vi "log analysis_gps.vi"() -> ()   [LabVIEW 2019] (continued)
\t-1.749398\t-175.069883\t0.291000\t0.008000\n\t\n15:47:23.2\tlog_raw\tgps_raw\t#INSPVAXA,USB3,0,49.5,FINESTEERING,2107,283661.200,02000000,471d,15824;INS_ALIGNMENT_COMPLETE,INS_RTKFIXED,37.37126187130,126.72202999654,7.8827,22.3000,0.0166,-0.2769,0.0144,-0.534535443,-1.728487239,265.001971487,0.4359,0.2961,0.5778,0.1123,0.0926,0.0785,0.0961,0.1008,5.1311,0f000001,0*51cc925f\n\tsystem status\tnormal 2 27.800000 0 0\trobot status\t105.841527\t125.597807\t7.882700\t-0.534535\t-1.728487\t-175.001971\t0.284000\t0.012000\n\t\n15:47:23.7\tlog_raw\tgps_raw\t#DUALANTENNAHEADINGA,USB3,0,49.5,FINESTEERING,2107,283661.700,02000000,d426,15824;INSUFFICIENT_OBS,NONE,-1.000000000,0.000000000,0.000000000,0.0,0.000000000,0.000000000,\"631T\",12,4,4,3,04,00,20,03*15f903f8\n\tsystem status\tnormal 2 27.800000 0 0\trobot status\t105.702965\t125.590854\t7.884200\t-0.871076\t-0.905355\t-174.823029\t0.389000\t-0.120000\n\t\n15:47:24.2\tlog_raw\tgps_raw\t#DUALANTENNAHEADINGA,USB3,0,48.0,FINESTEERING,2107,283662.200,02000000,d426,15824;INSUFFICIENT_OBS,NONE,-1.000000000,0.000000000,0.000000000,0.0,0.000000000,0.000000000,\"631T\",12,4,4,3,04,00,20,03*45bc2fa2\n\tsystem status\tnormal 2 27.800000 0 0\trobot status\t105.562658\t125.586822\t7.884400\t-0.819819\t-0.206414\t-174.816486\t0.286000\t0.006000\n\t\n15:47:24.7\tlog_raw\tgps_raw\t#INSPVAXA,USB3,0,48.0,FINESTEERING,2107,283662.700,02000000,471d,15824;INS_ALIGNMENT_COMPLETE,INS_RTKFIXED,37.37126171572,126.72202522799,7.8823,22.3000,-0.0067,-0.2635,0.0136,-1.179961552,0.094212856,265.044425368,0.4362,0.2961,0.5779,0.1131,0.0926,0.0785,0.0961,0.1008,5.1327,0f000001,0*9a1b8d6f\n\tsystem status\tnormal 2 27.900000 0 0\trobot status\t105.419137\t125.580546\t7.882300\t-1.179962\t0.094213\t-175.044425\t0.278000\t0.003000\n\t\n15:47:25.2\tlog_raw\tgps_raw\t#DUALANTENNAHEADINGA,USB3,0,49.0,FINESTEERING,2107,283663.200,02000000,d426,15824;INSUFFICIENT_OBS,NONE,-1.000000000,0.000000000,0.000000000,0.0,0.000000000,0.000000000,\"631T\",12,4,4,3,04,00,20,03*4c20fddf\n\tsystem status\tnormal 2 27.900000 0 0\trobot status\t105.284116\t125.575156\t7.883700\t-1.526473\t0.492436\t-175.160100\t0.292000\t-0.033000\n\t\n15:47:25.7\tlog_raw\tgps_raw\t#DUALANTENNAHEADINGA,USB3,0,49.0,FINESTEERING,2107,283663.700,02000000,d426,15824;INSUFFICIENT_OBS,NONE,-1.000000000,0.000000000,0.000000000,0.0,0.000000000,0.000000000,\"631T\",13,4,4,3,04,00,20,03*4cd16cde\n\tsystem status\tnormal 2 27.900000 0 0\trobot status\t105.149860\t125.571077\t7.886600\t-1.585695\t1.181553\t-175.183100\t0.294000\t-0.020000\n\t\n15:47:26.2\tlog_raw\tgps_raw\t#DUALANTENNAHEADINGA,USB3,0,53.0,FINESTEERING,2107,283664.200,02000000,d426,15824;INSUFFICIENT_OBS,NONE,-1.000000000,0.000000000,0.000000000,0.0,0.000000000,0.000000000,\"631T\",14,4,4,3,04,00,20,02*f110e9d9\n\tsystem status\tnormal 2 27.800000 0 0\trobot status\t105.010520\t125.564554\t7.892600\t-1.984977\t1.172369\t-175.175072\t0.296000\t-0.009000\n\t\n15:47:26.7\tlog_raw\tgps_raw\t#DUALANTENNAHEADINGA,USB3,0,53.0,FINESTEERING,2107,283664.700,02000000,d426,15824;INSUFFICIENT_OBS,NONE,-1.000000000,0.000000000,0.000000000,0.0,0.000000000,0.000000000,\"631T\",15,4,4,3,04,00,20,02*f1e178d8\n\tsystem status\tnormal 2 27.900000 0 0\trobot status\t104.866280\t125.562759\t7.898100\t-1.643568\t1.568433\t-175.385137\t0.303000\t-0.018000\n\t\n15:47:27.2\tlog_raw\tgps_raw\t#DUALANTENNAHEADINGA,USB3,0,50.0,FINESTEERING,2107,283665.200,02000000,d426,15824;INSUFFICIENT_OBS,NONE,-1.000000000,0.000000000,0.000000000,0.0,0.000000000,0.000000000,\"631T\",13,4,4,3,04,00,20,03*0d3c2d31\n\tsystem status\tnormal 2 27.900000 0 0\trobot status\t104.717899\t125.556202\t7.901900\t-2.175035\t2.158905\t-175.701482\t0.303000\t-0.049000\n\t\n15:47:27.7\tlog_raw\tgps_raw\t#DUALANTENNAHEADINGA,USB3,0,50.0,FINESTEERING,2107,283665.700,02000000,d426,15824;INSUFFICIENT_OBS,NONE,-1.000000000,0.000000000,0.000000000,0.0,0.000000000,0.000000000,\"631T\",12,4,4,3,04,00,20,02*7aca8ca6\n\tsystem status\tnormal 2 27.800000 0 0\trobot status\t104.573395\t125.553571\t7.908800\t-2.110560\t2.141372\t-176.036510\t0.311000\t-0.034000\n\t\n15:47:28.2\tlog_raw\tgps_raw\t#DUALANTENNAHEADINGA,USB3,0,49.5,FINESTEERING,2107,283666.200,02000000,d426,15824;INSUFFICIENT_OBS,NONE,-1.000000000,0.000000000,0.000000000,0.0,0.000000000,0.000000000,\"631T\",12,4,4,3,04,00,20,03*18930aef\n\tsystem status\tnormal 2 27.800000 0 0\trobot status\t104.418430\t125.550188\t7.915100\t-2.269862\t2.122656\t-176.495930\t0.394000\t0.113000\n\t\n15:47:28.7\tlog_raw\tgps_raw\t\tsystem status\tnormal 2 27.800000 0 0\trobot status\t104.271361\t125.550531\t7.920700\t-2.130480\t1.933923\t-177.098669\t0.402000\t0.141000\n\t\n15:47:29.2\tlog_raw\tgps_raw\t#DUALANTENNAHEADINGA,USB3,0,51.0,FINESTEERING,2107,283667.200,02000000,d426,15824;INSUFFICIENT_OBS,NONE,-1.000000000,0.000000000,0.000000000,0.0,0.000000000,0.000000000,\"631T\",14,4,4,3,04,00,20,03*f8f6796c\n\tsystem status\tnormal 2 27.700000 0 0\trobot status\t104.125597\t125.551980\t7.926900\t-2.197035\t1.911660\t-177.915300\t0.350000\t0.055000\n\t\n15:47:29.7\tlog_raw\tgps_raw\t#DUALANTENNAHEADINGA,USB3,0,51.0,FINESTEERING,2107,283667.700,02000000,d426,15824;INSUFFICIENT_OBS,NONE,-1.000000000,0.000000000,0.000000000,0.0,0.000000000,0.000000000,\"631T\",14,4,4,3,04,00,20,02*58e258a3\n\tsystem status\tnormal 2 27.700000 0 0\trobot status\t103.980327\t125.554709\t7.933500\t-2.393208\t1.875693\t-178.717408\t0.289000\t-0.036000\n\t\n15:47:30.2\tlog_raw\tgps_raw\t#DUALANTENNAHEADINGA,USB3,0,51.5,FINESTEERING,2107,283668.200,02000000,d426,15824;INSUFFICIENT_OBS,NONE,-1.000000000,0.000000000,0.000000000,0.0,0.000000000,0.000000000,\"631T\",13,4,4,3,04,00,20,03*e5e926ef\n\tsystem status\tnormal 2 27.800000 0 0\trobot status\t103.834212\t125.563002\t7.939200\t-2.024919\t1.603029\t-179.561928\t0.229000\t-0.114000\n\t\n15:47:30.7\tlog_raw\tgps_raw\t#DUALANTENNAHEADINGA,USB3,0,51.5,FINESTEERING,2107,283668.700,02000000,d426,15824;INSUFFICIENT_OBS,NONE,-1.000000000,0.000000000,0.000000000,0.0,0.000000000,0.000000000,\"631T\",12,4,4,3,04,00,20,03*e518b7ee\n\tsystem status\tnormal 2 27.800000 0 0\trobot status\t103.706860\t125.571273\t7.943700\t-1.912750\t1.464702\t179.878930\t0.099000\t-0.005000\n\t\n15:47:31.2\tlog_raw\tgps_raw\t#DUALANTENNAHEADINGA,USB3,0,49.0,FINESTEERING,2107,283669.200,02000000,d426,15824;INSUFFICIENT_OBS,NONE,-1.000000000,0.000000000,0.000000000,0.0,0.000000000,0.000000000,\"631T\",12,4,4,3,04,00,20,03*4fb2de27\n\tsystem status\tnormal 2 27.800000 0 0\trobot status\t103.578139\t125.580373\t7.945800\t-2.015025\t1.317294\t179.548370\t0.270000\t-0.089000\n\t\n15:47:31.7\tlog_raw\tgps_raw\t#DUALANTENNAHEADINGA,USB3,0,49.0,FINESTEERING,2107,283669.700,02000000,d426,15824;INSUFFICIENT_OBS,NONE,-1.000000000,0.000000000,0.000000000,0.0,0.000000000,0.000000000,\"631T\",12,4,4,3,04,00,20,02*efa6ffe8\n\tsystem status\tnormal 2 27.800000 0 0\trobot status\t103.443389\t125.589391\t7.947800\t-2.168646\t1.038797\t179.383085\t0.315000\t0.000000\n\t\n15:47:32.2\tlog_raw\tgps_raw\t#DUALANTENNAHEADINGA,USB3,0,50.0,FINESTEERING,2107,283670.200,02000000,d426,15824;INSUFFICIENT_OBS,NONE,-1.000000000,0.000000000,0.000000000,0.0,0.000000000,0.000000000,\"631T\",12,4,4,3,04,00,20,03*24750ee1\n\tsystem status\tnormal 2 27.800000 0 0\trobot status\t103.309611\t125.601920\t7.951600\t-1.888949\t0.915016\t179.178170\t0.304000\t0.012000\n\t\n15:47:32.7\tlog_raw\tgps_raw\t#DUALANTENNAHEADINGA,USB3,0,50.0,FINESTEERING,2107,283670.700,02000000,d426,15824;INSUFFICIENT_OBS,NONE,-1.000000000,0.000000000,0.000000000,0.0,0.000000000,0.000000000,\"631T\",13,4,4,3,04,00,20,03*24849fe0\n\tsystem status\tnormal 2 27.900000 0 0\trobot status\t103.174226\t125.616514\t7.954700\t-1.437536\t0.949843\t179.107263\t0.291000\t0.026000\n\t\n15:47:33.2\tlog_raw\tgps_raw\t#DUALANTENNAHEADINGA,USB3,0,50.0,FINESTEERING,2107,283671.200,02000000,d426,15824;INSUFFICIENT_OBS,NONE,-1.000000000,0.000000000,0.000000000,0.0,0.000000000,0.000000000,\"631T\",13,4,4,3,04,00,20,02*e948baf6\n\tsystem status\tnormal 2 27.800000 0 0\trobot status\t103.027425\t125.628258\t7.958900\t-1.451100\t0.751950\t179.111320\t0.296000\t0.032000\n\t\n15:47:33.7\tlog_raw\tgps_raw\t#DUALANTENNAHEADINGA,USB3,0,50.0,FINESTEERING,2107,283671.700,02000000,d426,15824;INSUFFICIENT_OBS,NONE,-1.000000000,0.000000000,0.000000000,0.0,0.000000000,0.000000000,\"631T\",12,4,4,3,04,00,20,02*e9b92bf7\n\tsystem status\tnormal 2 27.900000 0 0\trobot status\t102.871613\t125.638877\t7.960600\t-1.577622\t0.823494\t179.153845\t0.306000\t0.029000\n\t\n15:47:34.2\tlog_raw\tgps_raw\t#DUALANTENNAHEADINGA,USB3,0,47.5,FINESTEERING,2107,283672.200,02000000,d426,15824;INSUFFICIENT_OBS,NONE,-1.000000000,0.000000000,0.000000000,0.0,0.000000000,0.000000000,\"631T\",13,4,4,3,04,00,20,03*4a2d65dd\n\tsystem status\tnormal 2 27.800000 0 0\trobot status\t102.727478\t125.652101\t7.963400\t-1.336233\t0.876198\t179.513411\t0.340000\t-0.041000\n\t\n15:47:34.7\tlog_raw\tgps_raw\t#DUALANTENNAHEADINGA,USB3,0,47.5,FINESTEERING,2107,283672.700,02000000,d426,15824;INSUFFICIENT_OBS,NONE,-1.000000000,0.000000000,0.000000000,0.0,0.000000000,0.000000000,\"631T\",11,4,4,3,04,00,20,03*e98a7275\n\tsystem status\tnormal 2 27.700000 0 0\trobot status\t102.584118\t125.664970\t7.965600\t-1.001130\t0.865934\t-179.684360\t0.289000\t0.047000\n\t\n15:47:35.2\tlog_raw\tgps_raw\t#DUALANTENNAHEADINGA,USB3,0,49.0,FINESTEERING,2107,283673.200,02000000,d426,15824;INSUFFICIENT_OBS,NONE,-1.000000000,0.000000000,0.000000000,0.0,0.000000000,0.000000000,\"631T\",12,4,4,3,04,00,20,02*c4457f3d\n\tsystem status\tnormal 2 27.500000 0 0\trobot status\t102.442950\t125.672792\t7.967600\t-1.200080\t0.869619\t-178.506958\t0.290000\t0.033000\n\t\n15:47:35.7\tlog_raw\tgps_raw\t#DUALANTENNAHEADINGA,USB3,0,49.0,FINESTEERING,2107,283673.700,02000000,d426,15824;INSUFFICIENT_OBS,NONE,-1.000000000,0.000000000,0.000000000,0.0,0.000000000,0.000000000,\"631T\",13,4,4,3,04,00,20,03*b3b3deaa\n\tsystem status\tnormal 2 27.400000 0 0\trobot status\t102.301599\t125.675630\t7.970100\t-1.366627\t0.503237\t-176.945977\t0.292000\t0.049000\n\t\n15:47:36.2\tlog_raw\tgps_raw\t#DUALANTENNAHEADINGA,USB3,0,50.0,FINESTEERING,2107,283674.200,02000000,d426,15824;INSUFFICIENT_OBS,NONE,-1.000000000,0.000000000,0.000000000,0.0,0.000000000,0.000000000,\"631T\",13,4,4,3,04,00,20,03*9f869b9c\n\tsystem status\tnormal 2 27.400000 0 0\trobot status\t102.163674\t125.676713\t7.974400\t-1.299675\t0.317092\t-175.226146\t0.304000\t0.058000\n\t\n15:47:36.7\tlog_raw\tgps_raw\t#INSPVAXA,USB3,0,50.0,FINESTEERING,2107,283674.750,02000000,471d,15824;INS_ALIGNMENT_COMPLETE,INS_RTKFIXED,37.37126252882,126.72198672229,7.9795,22.3000,-0.0186,-0.2998,0.0327,-1.236759140,0.298585225,263.242315357,0.4398,0.2975,0.5789,0.1131,0.0929,0.0786,0.0960,0.1008,5.0828,0f000001,0*30bc741b\n\tsystem status\tnormal 2 27.400000 0 0\trobot status\t102.008365\t125.670829\t7.979500\t-1.236759\t0.298585\t-173.242315\t0.310000\t0.068000\n\t\n15:47:37.2\tlog_raw\tgps_raw\t#DUALANTENNAHEADINGA,USB3,0,47.5,FINESTEERING,2107,283675.200,02000000,d426,15824;INSUFFICIENT_OBS,NONE,-1.000000000,0.000000000,0.000000000,0.0,0.000000000,0.000000000,\"631T\",12,4,4,3,04,00,20,02*30b1cd5d\n\tsystem status\tnormal 2 27.500000 0 0\trobot status\t101.881157\t125.662058\t7.983600\t-1.357425\t0.105413\t-171.884770\t0.302000\t0.058000\n\t\n15:47:37.7\tlog_raw\tgps_raw\t#DUALANTENNAHEADINGA,USB3,0,47.5,FINESTEERING,2107,283675.700,02000000,d426,15824;INSUFFICIENT_OBS,NONE,-1.000000000,0.000000000,0.000000000,0.0,0.000000000,0.000000000,\"631T\",13,4,4,3,04,00,20,03*47476cca\n\tsystem status\tnormal 2 27.500000 0 0\trobot status\t101.741807\t125.649863\t7.985900\t-1.401248\t0.156405\t-170.535957\t0.300000\t0.034000\n\t\n15:47:38.2\tlog_raw\tgps_raw\t#DUALANTENNAHEADINGA,USB3,0,50.0,FINESTEERING,2107,283676.200,02000000,d426,15824;INSUFFICIENT_OBS,NONE,-1.000000000,0.000000000,0.000000000,0.0,0.000000000,0.000000000,\"631T\",13,4,4,3,04,00,20,02*3331a2b8\n\tsystem status\tnormal 2 27.500000 0 0\trobot status\t101.602528\t125.635550\t7.989300\t-1.281281\t0.182913\t-169.273550\t0.304000\t0.035000\n\t\n15:47:38.7\tlog_raw\tgps_raw\t#INSPVAXA,USB3,0,50.0,FINESTEERING,2107,283676.750,02000000,471d,15824;INS_ALIGNMENT_COMPLETE,INS_RTKFIXED,37.37126202802,126.72198037867,7.9931,22.3000,-0.0270,-0.2983,0.0289,-1.276938431,0.174085147,258.154591337,0.4371,0.2976,0.5788,0.1128,0.0927,0.0785,0.0959,0.1007,5.0828,0f000001,0*1eb9a34f\n\tsystem status\tnormal 2 27.500000 0 0\trobot status\t101.446458\t125.615255\t7.993100\t-1.276938\t0.174085\t-168.154591\t0.309000\t0.036000\n\t\n15:47:39.2\tlog_raw\tgps_raw\t#INSPVAXA,USB3,0,47.5,FINESTEERING,2107,283677.250,02000000,471d,15824;INS_ALIGNMENT_COMPLETE,INS_RTKFIXED,37.37126184306,126.72197878066,7.9954,22.3000,-0.0249,-0.2800,0.0095,-1.329008924,0.068233484,257.455385518,0.4363,0.2976,0.5789,0.1128,0.0926,0.0785,0.0959,0.1006,5.0823,0f000001,0*a0488656\n\tsystem status\tnormal 2 27.700000 0 0\trobot status\t101.304909\t125.594729\t7.995400\t-1.329009\t0.068233\t-167.455386\t0.294000\t0.024000\n\t\n15:47:39.7\tlog_raw\tgps_raw\t\tsystem status\tnormal 2 27.700000 0 0\trobot status\t101.178617\t125.576497\t7.997000\t-1.321443\t0.121377\t-166.935462\t0.272000\t0.053000\n\t\n15:47:40.2\tlog_raw\tgps_raw\t\tsystem status\tnormal 2 27.600000 0 0\trobot status\t101.060799\t125.559123\t7.999900\t-1.339962\t0.318685\t-166.437151\t0.256000\t0.107000\n\t\n15:47:40.7\tlog_raw\tgps_raw\t#INSPVAXA,USB3,0,44.5,FINESTEERING,2107,283678.750,02000000,471d,15824;INS_ALIGNMENT_COMPLETE,INS_RTKFIXED,37.37126126052,126.72197417876,8.0025,22.3000,-0.0388,-0.3139,0.0075,-1.341441151,0.143163163,255.994609032,0.4352,0.2975,0.5790,0.1123,0.0928,0.0785,0.0959,0.1006,5.0816,0f000001,0*2dcb75ae\n\tsystem status\tnormal 2 27.700000 0 0\trobot status\t100.897280\t125.530081\t8.002500\t-1.341441\t0.143163\t-165.994609\t0.230000\t0.123000\n\t\n15:47:41.2\tlog_raw\tgps_raw\t#INSPVAXA,USB3,0,50.0,FINESTEERING,2107,283679.250,02000000,471d,15824;INS_ALIGNMENT_COMPLETE,INS_RTKFIXED,37.37126102386,126.72197256335,8.0029,22.3000,-0.0378,-0.3051,0.0239,-1.252291621,0.317106039,255.710782643,0.4355,0.2977,0.5792,0.1125,0.0927,0.0786,0.0959,0.1006,5.0819,0f000001,0*497f861f\n\tsystem status\tnormal 2 27.800000 0 0\trobot status\t100.754189\t125.503817\t8.002900\t-1.252292\t0.317106\t-165.710783\t0.206000\t0.142000\n\t\n15:47:41.7\tlog_raw\tgps_raw\t#DUALANTENNAHEADINGA,USB3,0,50.0,FINESTEERING,2107,283679.700,02000000,d426,15824;INSUFFICIENT_OBS,NONE,-1.000000000,0.000000000,0.000000000,0.0,0.000000000,0.000000000,\"631T\",13,4,4,3,04,00,20,03*917eb173\n\tsystem status\tnormal 2 27.800000 0 0\trobot status\t100.626127\t125.478833\t8.004200\t-1.300155\t0.357436\t-165.554866\t0.246000\t0.082000\n\t\n15:47:42.2\tlog_raw\tgps_raw\t#INSPVAXA,USB3,0,49.5,FINESTEERING,2107,283680.250,02000000,471d,15824;INS_ALIGNMENT_COMPLETE,INS_RTKFIXED,37.37126052998,126.72196935056,8.0055,22.3000,-0.0369,-0.2979,0.0271,-1.221523222,0.248269535,255.390291305,0.4350,0.2975,0.5791,0.1126,0.0927,0.0786,0.0959,0.1006,5.0824,0f000001,0*4c9222e8\n\tsystem status\tnormal 2 27.800000 0 0\trobot status\t100.469606\t125.449008\t8.005500\t-1.221523\t0.248270\t-165.390291\t0.265000\t0.060000\n\t\n15:47:42.7\tlog_raw\tgps_raw\t#INSPVAXA,USB3,0,49.5,FINESTEERING,2107,283680.750,02000000,471d,15824;INS_ALIGNMENT_COMPLETE,INS_RTKFIXED,37.37126029067,126.72196774054,8.0075,22.3000,-0.0484,-0.2930,0.0156,-1.123777574,0.215686141,255.306454627,0.4350,0.2975,0.5791,0.1126,0.0927,0.0786,0.0959,0.1006,5.0824,0f000001,0*b1d08eab\n\tsystem status\tnormal 2 27.800000 0 0\trobot status\t100.326993\t125.422450\t8.007500\t-1.123778\t0.215686\t-165.306455\t0.353000\t-0.070000\n\t\n15:47:43.2\tlog_raw\tgps_raw\t#DUALANTENNAHEADINGA,USB3,0,47.5,FINESTEERING,2107,283681.200,02000000,d426,15824;INSUFFICIENT_OBS,NONE,-1.000000000,0.000000000,0.000000000,0.0,0.000000000,0.000000000,\"631T\",13,4,4,3,04,00,20,02*8c2dc70b\n\tsystem status\tnormal 2 27.800000 0 0\trobot status\t100.200318\t125.396716\t8.008600\t-1.364227\t0.259230\t-165.309745\t0.296000\t0.001000\n\t\n15:47:43.7\tlog_raw\tgps_raw\t#DUALANTENNAHEADINGA,USB3,0,47.5,FINESTEERING,2107,283681.700,02000000,d426,15824;INSUFFICIENT_OBS,NONE,-1.000000000,0.000000000,0.000000000,0.0,0.000000000,0.000000000,\"631T\",13,4,4,3,04,00,20,03*2c39e6c4\n\tsystem status\tnormal 2 27.800000 0 0\trobot status\t100.058386\t125.369198\t8.010200\t-1.337236\t0.106302\t-165.240050\t0.349000\t-0.071000\n\t\n15:47:44.2\tlog_raw\tgps_raw\t#DUALANTENNAHEADINGA,USB3,0,53.0,FINESTEERING,2107,283682.200,02000000,d426,15824;INSUFFICIENT_OBS,NONE,-1.000000000,0.000000000,0.000000000,0.0,0.000000000,0.000000000,\"631T\",13,4,4,3,04,00,20,02*f482535a\n\tsystem status\tnormal 2 27.800000 0 0\trobot status\t99.916585\t125.340598\t8.012100\t-1.398981\t0.149147\t-165.140056\t0.293000\t0.019000\n\t\n15:47:44.7\tlog_raw\tgps_raw\t#INSPVAXA,USB3,0,53.0,FINESTEERING,2107,283682.750,02000000,471d,15824;INS_ALIGNMENT_COMPLETE,INS_RTKFIXED,37.37125926494,126.72196137618,8.0142,22.3000,-0.0531,-0.2940,0.0193,-1.467222683,0.192661373,255.088191975,0.4346,0.2973,0.5792,0.1126,0.0928,0.0786,0.0959,0.1005,5.0834,0f000001,0*e49cbeff\n\tsystem status\tnormal 2 27.800000 0 0\trobot status\t99.763248\t125.308616\t8.014200\t-1.467223\t0.192661\t-165.088192\t0.352000\t-0.079000\n\t\n15:47:45.2\tlog_raw\tgps_raw\t#DUALANTENNAHEADINGA,USB3,0,51.5,FINESTEERING,2107,283683.200,02000000,d426,15824;INSUFFICIENT_OBS,NONE,-1.000000000,0.000000000,0.000000000,0.0,0.000000000,0.000000000,\"631T\",13,4,4,3,04,00,20,03*73ae2c91\n\tsystem status\tnormal 2 27.800000 0 0\trobot status\t99.634729\t125.283250\t8.015500\t-1.390828\t0.179060\t-165.064944\t0.292000\t0.016000\n\t\n15:47:45.7\tlog_raw\tgps_raw\t#INSPVAXA,USB3,0,51.5,FINESTEERING,2107,283683.750,02000000,471d,15824;INS_ALIGNMENT_COMPLETE,INS_RTKFIXED,37.37125874592,126.72195815928,8.0147,22.3000,-0.0440,-0.2967,0.0132,-1.341050050,-0.067435832,254.924614252,0.4345,0.2971,0.5791,0.1126,0.0928,0.0785,0.0959,0.1005,5.0840,0f000001,0*701f89f0\n\tsystem status\tnormal 2 27.800000 0 0\trobot status\t99.478300\t125.251016\t8.014700\t-1.341050\t-0.067436\t-164.924614\t0.429000\t-0.182000\n\t\n15:47:46.2\tlog_raw\tgps_raw\t#DUALANTENNAHEADINGA,USB3,0,52.0,FINESTEERING,2107,283684.200,02000000,d426,15824;INSUFFICIENT_OBS,NONE,-1.000000000,0.000000000,0.000000000,0.0,0.000000000,0.000000000,\"631T\",13,4,4,3,04,00,20,02*27679969\n\tsystem status\tnormal 2 27.800000 0 0\trobot status\t99.351672\t125.225493\t8.015100\t-1.339484\t-0.170891\t-164.827826\t0.237000\t0.097000\n\t\n15:47:46.7\tlog_raw\tgps_raw\t#INSPVAXA,USB3,0,52.0,FINESTEERING,2107,283684.750,02000000,471d,15824;INS_ALIGNMENT_COMPLETE,INS_RTKFIXED,37.37125823226,126.72195499542,8.0159,22.3000,-0.0425,-0.2912,0.0233,-1.481512417,-0.232627459,254.717814630,0.4345,0.2970,0.5790,0.1126,0.0928,0.0785,0.0959,0.1005,5.0847,0f000001,0*bc004070\n\tsystem status\tnormal 2 27.800000 0 0\trobot status\t99.198051\t125.194011\t8.015900\t-1.481512\t-0.232627\t-164.717815\t0.430000\t-0.193000\n\t\n15:47:47.2\tlog_raw\tgps_raw\t#DUALANTENNAHEADINGA,USB3,0,54.0,FINESTEERING,2107,283685.200,02000000,d426,15824;INSUFFICIENT_OBS,NONE,-1.000000000,0.000000000,0.000000000,0.0,0.000000000,0.000000000,\"631T\",13,4,4,3,04,00,20,03*bf535cbf\n\tsystem status\tnormal 2 27.800000 0 0\trobot status\t99.072052\t125.168405\t8.017800\t-1.521026\t-0.355699\t-164.511817\t0.245000\t0.084000\n\t\n15:47:47.7\tlog_raw\tgps_raw\t#DUALANTENNAHEADINGA,USB3,0,54.0,FINESTEERING,2107,283685.700,02000000,d426,15824;INSUFFICIENT_OBS,NONE,-1.000000000,0.000000000,0.000000000,0.0,0.000000000,0.000000000,\"631T\",15,4,4,3,04,00,20,03*f59c46f5\n\tsystem status\tnormal 2 27.800000 0 0\trobot status\t98.933125\t125.139867\t8.018400\t-1.376883\t-0.262136\t-164.273849\t0.254000\t0.072000\n\t\n15:47:48.2\tlog_raw\tgps_raw\t#INSPVAXA,USB3,0,47.0,FINESTEERING,2107,283686.250,02000000,471d,15824;INS_ALIGNMENT_COMPLETE,INS_RTKFIXED,37.37125745168,126.72195028422,8.0177,22.3000,-0.0421,-0.2788,0.0295,-1.327379585,-0.197998940,254.015433265,0.4342,0.2970,0.5788,0.1125,0.0928,0.0785,0.0959,0.1004,5.0859,0f000001,0*059a606c\n\tsystem status\tnormal 2 27.800000 0 0\trobot status\t98.780741\t125.107384\t8.017700\t-1.327380\t-0.197999\t-164.015433\t0.374000\t-0.106000\n\t\n15:47:48.7\tlog_raw\tgps_raw\t#INSPVAXA,USB3,0,47.0,FINESTEERING,2107,283686.750,02000000,471d,15824;INS_ALIGNMENT_COMPLETE,INS_RTKFIXED,37.37125719652,126.72194873669,8.0201,22.3000,-0.0424,-0.2865,0.0311,-1.155721868,-0.143426026,253.623399398,0.4342,0.2970,0.5788,0.1125,0.0928,0.0785,0.0959,0.1004,5.0859,0f000001,0*874a06ff\n\tsystem status\tnormal 2 27.800000 0 0\trobot status\t98.643663\t125.079067\t8.020100\t-1.155722\t-0.143426\t-163.623399\t0.285000\t0.042000\n\t\n15:47:49.2\tlog_raw\tgps_raw\t#INSPVAXA,USB3,0,48.5,FINESTEERING,2107,283687.250,02000000,471d,15824;INS_ALIGNMENT_COMPLETE,INS_RTKFIXED,37.37125692308,126.72194717786,8.0216,22.3000,-0.0335,-0.2418,0.0315,-1.192319582,-0.154191109,253.231237079,0.4341,0.2971,0.5788,0.1124,0.0928,0.0785,0.0959,0.1004,5.0866,0f000001,0*54818d56\n\tsystem status\tnormal 2 27.700000 0 0\trobot status\t98.505584\t125.048721\t8.021600\t-1.192320\t-0.154191\t-163.231237\t0.319000\t-0.041000\n\t\n15:47:49.7\tlog_raw\tgps_raw\t\tsystem status\tnormal 2 27.700000 0 0\trobot status\t98.411193\t125.029187\t8.022300\t-1.203648\t0.044720\t-163.074738\t0.395000\t-0.024000\n\t\n15:47:50.2\tlog_raw\tgps_raw\t#INSPVAXA,USB3,0,48.0,FINESTEERING,2107,283688.250,02000000,471d,15824;INS_ALIGNMENT_COMPLETE,INS_RTKFIXED,37.37125642172,126.72194437677,8.0235,22.3000,-0.0500,-0.3046,0.0059,-1.164662178,-0.014385646,252.588332690,0.4343,0.2973,0.5789,0.1124,0.0928,0.0785,0.0959,0.1004,5.0876,0f000001,0*78a62f40\n\tsystem status\tnormal 2 27.700000 0 0\trobot status\t98.257468\t124.993080\t8.023500\t-1.164662\t-0.014386\t-162.588333\t0.345000\t-0.033000\n\t\n15:47:50.7\tlog_raw\tgps_raw\t#INSPVAXA,USB3,0,48.0,FINESTEERING,2107,283688.750,02000000,471d,15824;INS_ALIGNMENT_COMPLETE,INS_RTKFIXED,37.37125610282,126.72194283979,8.0244,22.3000,-0.0543,-0.2923,0.0224,-1.111219856,-0.008949492,252.070206998,0.4343,0.2973,0.5789,0.1124,0.0928,0.0785,0.0959,0.1004,5.0876,0f000001,0*c44a5f5d\n\tsystem status\tnormal 2 27.700000 0 0\trobot status\t98.121325\t124.957689\t8.024400\t-1.111220\t-0.008949\t-162.070207\t0.361000\t-0.068000\n\t\n15:47:51.2\tlog_raw\tgps_raw\t#INSPVAXA,USB3,0,50.0,FINESTEERING,2107,283689.250,02000000,471d,15824;INS_ALIGNMENT_COMPLETE,INS_RTKFIXED,37.37125577091,126.72194129043,8.0250,22.3000,-0.0553,-0.2846,0.0299,-1.126484070,-0.034453614,251.571777713,0.4347,0.2976,0.5789,0.1123,0.0927,0.0785,0.0959,0.1004,5.0890,0f000001,0*4752c184\n\tsystem status\tnormal 2 27.800000 0 0\trobot status\t97.984085\t124.920853\t8.025000\t-1.126484\t-0.034454\t-161.571778\t0.264000\t0.067000\n\t\n15:47:51.7\tlog_raw\tgps_raw\t#INSPVAXA,USB3,0,50.0,FINESTEERING,2107,283689.750,02000000,471d,15824;INS_ALIGNMENT_COMPLETE,INS_RTKFIXED,37.37125543079,126.72193970784,8.0254,22.3000,-0.0623,-0.2845,0.0344,-1.115085970,-0.181471482,251.113733002,0.4347,0.2976,0.5789,0.1123,0.0927,0.0785,0.0959,0.1004,5.0890,0f000001,0*e6043553\n\tsystem status\tnormal 2 27.700000 0 0\trobot status\t97.843902\t124.883107\t8.025400\t-1.115086\t-0.181471\t-161.113733\t0.347000\t-0.040000\n\t\n15:47:52.2\tlog_raw\tgps_raw\t#INSPVAXA,USB3,0,51.5,FINESTEERING,2107,283690.250,02000000,471d,15824;INS_ALIGNMENT_COMPLETE,INS_RTKFIXED,37.37125508435,126.72193816260,8.0268,22.3000,-0.0829,-0.2745,0.0314,-1.131096634,-0.362526816,250.672431743,0.4348,0.2977,0.5789,0.1123,0.0927,0.0785,0.0959,0.1004,5.0905,0f000001,0*0f3c6f4d\n\tsystem status\tnormal 2 27.700000 0 0\trobot status\t97.707027\t124.844659\t8.026800\t-1.131097\t-0.362527\t-160.672432\t0.294000\t0.018000\n\t\n15:47:52.7\tlog_raw\tgps_raw\t#INSPVAXA,USB3,0,51.5,FINESTEERING,2107,283690.750,02000000,471d,15824;INS_ALIGNMENT_COMPLETE,INS_RTKFIXED,37.37125472381,126.72193660268,8.0270,22.3000,-0.0761,-0.2693,0.0189,-1.124428932,-0.555258111,250.148936400,0.4348,0.2977,0.5789,0.1123,0.0927,0.0785,0.0959,0.1004,5.0905,0f000001,0*bccc2e0c\n\tsystem status\tnormal 2 27.700000 0 0\trobot status\t97.568852\t124.804646\t8.027000\t-1.124429\t-0.555258\t-160.148936\t0.283000\t0.041000\n\t\n15:47:53.2\tlog_raw\tgps_raw\t#INSPVAXA,USB3,0,51.0,FINESTEERING,2107,283691.250,02000000,471d,15824;INS_ALIGNMENT_COMPLETE,INS_RTKFIXED,37.37125435874,126.72193505456,8.0263,22.3000,-0.0670,-0.2696,0.0092,-1.064456242,-0.547416950,249.737681282,0.4347,0.2977,0.5789,0.1123,0.0927,0.0785,0.0959,0.1004,5.0921,0f000001,0*f2a7f55d\n\tsystem status\tnormal 2 27.700000 0 0\trobot status\t97.431722\t124.764131\t8.026300\t-1.064456\t-0.547417\t-159.737681\t0.301000\t-0.002000\n\t\n15:47:53.7\tlog_raw\tgps_raw\t#INSPVAXA,USB3,0,51.0,FINESTEERING,2107,283691.750,02000000,471d,15824;INS_ALIGNMENT_COMPLETE,INS_RTKFIXED,37.37125397017,126.72193349362,8.0255,22.3000,-0.0691,-0.2936,0.0158,-1.034003666,-0.605283129,249.246949956,0.4347,0.2977,0.5789,0.1123,0.0927,0.0785,0.0959,0.1004,5.0921,0f000001,0*27b79f83\n\tsystem status\tnormal 2 27.700000 0 0\trobot status\t97.293457\t124.721007\t8.025500\t-1.034004\t-0.605283\t-159.246950\t0.247000\t0.099000\n\t\n15:47:54.2\tlog_raw\tgps_raw\t#INSPVAXA,USB3,0,52.0,FINESTEERING,2107,283692.250,02000000,471d,15824;INS_ALIGNMENT_COMPLETE,INS_RTKFIXED,37.37125358988,126.72193199872,8.0234,22.3000,-0.0664,-0.2884,0.0105,-1.029506848,-0.448748893,248.703805210,0.4344,0.2976,0.5789,0.1123,0.0927,0.0785,0.0960,0.1004,5.0936,0f000001,0*b0abd4b9\n\tsystem status\tnormal 2 27.700000 0 0\trobot status\t97.161041\t124.678802\t8.023400\t-1.029507\t-0.448749\t-158.703805\t0.229000\t0.121000\n\t\n15:47:54.7\tlog_raw\tgps_raw\t#INSPVAXA,USB3,0,52.0,FINESTEERING,2107,283692.750,02000000,471d,15824;INS_ALIGNMENT_COMPLETE,INS_RTKFIXED,37.37125319556,126.72193048668,8.0218,22.3000,-0.0721,-0.2829,0.0182,-0.873709041,-0.554913446,248.258505340,0.4344,0.2976,0.5789,0.1123,0.0927,0.0785,0.0960,0.1004,5.0936,0f000001,0*33541c24\n\tsystem status\tnormal 2 27.700000 0 0\trobot status\t97.027107\t124.635040\t8.021800\t-0.873709\t-0.554913\t-158.258505\t0.387000\t-0.130000\n\t\n15:47:55.2\tlog_raw\tgps_raw\t#INSPVAXA,USB3,0,52.0,FINESTEERING,2107,283693.250,02000000,471d,15824;INS_ALIGNMENT_COMPLETE,INS_RTKFIXED,37.37125278430,126.72192895782,8.0198,22.3000,-0.0808,-0.2833,0.0124,-0.750595920,-0.512604817,247.887825209,0.4345,0.2977,0.5790,0.1123,0.0927,0.0785,0.0960,0.1005,5.0951,0f000001,0*33503232\n\tsystem status\tnormal 2 27.700000 0 0\trobot status\t96.891683\t124.589398\t8.019800\t-0.750596\t-0.512605\t-157.887825\t0.301000\t0.008000\n\t\n15:47:55.7\tlog_raw\tgps_raw\t#INSPVAXA,USB3,0,52.0,FINESTEERING,2107,283693.750,02000000,471d,15824;INS_ALIGNMENT_COMPLETE,INS_RTKFIXED,37.37125237385,126.72192745643,8.0181,22.3000,-0.0699,-0.2766,0.0107,-0.708441706,-0.569028922,247.469165126,0.4345,0.2977,0.5790,0.1123,0.0927,0.0785,0.0960,0.1005,5.0951,0f000001,0*b12f53f8\n\tsystem status\tnormal 2 27.700000 0 0\trobot status\t96.758692\t124.543846\t8.018100\t-0.708442\t-0.569029\t-157.469165\t0.271000\t0.056000\n\t\n15:47:56.2\tlog_raw\tgps_raw\t#INSPVAXA,USB3,0,51.5,FINESTEERING,2107,283694.250,02000000,471d,15824;INS_ALIGNMENT_COMPLETE,INS_RTKFIXED,37.37125195619,126.72192597903,8.0151,22.3000,-0.0814,-0.2811,0.0110,-0.711365496,-0.463120250,247.118464084,0.4343,0.2979,0.5790,0.1123,0.0927,0.0785,0.0960,0.1005,5.0966,0f000001,0*fc596ab1\n\tsystem status\tnormal 2 27.700000 0 0\trobot status\t96.627827\t124.497494\t8.015100\t-0.711365\t-0.463120\t-157.118464\t0.244000\t0.090000\n\t\n15:47:56.7\tlog_raw\tgps_raw\t#INSPVAXA,USB3,0,51.5,FINESTEERING,2107,283694.750,02000000,471d,15824;INS_ALIGNMENT_COMPLETE,INS_RTKFIXED,37.37125151893,126.72192448231,8.0119,22.3000,-0.0800,-0.2663,0.0091,-0.771660159,-0.376939407,246.768281160,0.4343,0.2979,0.5790,0.1123,0.0927,0.0785,0.0960,0.1005,5.0966,0f000001,0*6d22b1be\n\tsystem status\tnormal 2 27.800000 0 0\trobot status\t96.495250\t124.448966\t8.011900\t-0.771660\t-0.376939\t-156.768281\t0.201000\t0.145000\n\t\n15:47:57.2\tlog_raw\tgps_raw\t#INSPVAXA,USB3,0,48.0,FINESTEERING,2107,283695.250,02000000,471d,15824;INS_ALIGNMENT_COMPLETE,INS_RTKFIXED,37.37125106123,126.72192297885,8.0100,22.3000,-0.0761,-0.2505,0.0231,-0.897100380,-0.291610583,246.370264659,0.4345,0.2982,0.5790,0.1123,0.0927,0.0785,0.0960,0.1005,5.0981,0f000001,0*3984aa9f\n\tsystem status\tnormal 2 27.700000 0 0\trobot status\t96.362076\t124.398170\t8.010000\t-0.897100\t-0.291611\t-156.370265\t0.326000\t-0.030000\n\t\n15:47:57.7\tlog_raw\tgps_raw\t#INSPVAXA,USB3,0,48.0,FINESTEERING,2107,283695.750,02000000,471d,15824;INS_ALIGNMENT_COMPLETE,INS_RTKFIXED,37.37125059397,126.72192150260,8.0095,22.3000,-0.0806,-0.2555,0.0180,-1.082975458,-0.280956917,246.024954508,0.4345,0.2982,0.5790,0.1123,0.0927,0.0785,0.0960,0.1005,5.0981,0f000001,0*61086754\n\tsystem status\tnormal 2 27.700000 0 0\trobot status\t96.231312\t124.346313\t8.009500\t-1.082975\t-0.280957\t-156.024955\t0.340000\t-0.049000\n\t\n15:47:58.2\tlog_raw\tgps_raw\t#INSPVAXA,USB3,0,48.5,FINESTEERING,2107,283696.250,02000000,471d,15824;INS_ALIGNMENT_COMPLETE,INS_RTKFIXED,37.37125013310,126.72192002149,8.0081,22.3000,-0.0880,-0.2655,0.0330,-1.084281837,-0.279647129,245.685810619,0.4346,0.2982,0.5792,0.1123,0.0927,0.0785,0.0960,0.1005,5.0996,0f000001,0*ddc3e251\n\tsystem status\tnormal 2 27.700000 0 0\trobot status\t96.100117\t124.295165\t8.008100\t-1.084282\t-0.279647\t-155.685811\t0.417000\t-0.156000\n\t\n15:47:58.7\tlog_raw\tgps_raw\t#INSPVAXA,USB3,0,48.5,FINESTEERING,2107,283696.750,02000000,471d,15824;INS_ALIGNMENT_COMPLETE,INS_RTKFIXED,37.37124978634,126.72191884253,8.0066,22.3000,0.0400,0.0236,0.0167,-1.049670935,-0.308268923,245.402478860,0.4346,0.2982,0.5792,0.1123,0.0927,0.0785,0.0960,0.1005,5.0996,0f000001,0*5343d95d\n\tsystem status\tnormal 2 27.800000 0 0\trobot status\t95.995687\t124.256681\t8.006600\t-1.049671\t-0.308269\t-155.402479\t0.058000\t0.016000\n\t\n15:47:59.2\tlog_raw\tgps_raw\t#INSPVAXA,USB3,0,49.5,FINESTEERING,2107,283697.250,02000000,471d,15824;INS_ALIGNMENT_COMPLETE,INS_RTKFIXED,37.37124936191,126.72191751580,8.0075,22.3000,-0.0790,-0.2224,0.0305,-1.160332211,-0.255386119,245.257033584,0.4348,0.2981,0.5792,0.1123,0.0927,0.0785,0.0960,0.1005,5.1012,0f000001,0*9bb241a9\n\tsystem status\tnormal 2 27.800000 0 0\trobot status\t95.878168\t124.209578\t8.007500\t-1.160332\t-0.255386\t-155.257034\t0.328000\t0.026000\n\t\n15:47:59.7\tlog_raw\tgps_raw\t#INSPVAXA,USB3,0,49.5,FINESTEERING,2107,283697.750,02000000,471d,15824;INS_ALIGNMENT_COMPLETE,INS_RTKFIXED,37.37124887882,126.72191610954,8.0072,22.3000,-0.0796,-0.2609,0.0250,-1.450872911,-0.189081024,245.072886035,0.4348,0.2981,0.5792,0.1123,0.0927,0.0785,0.0960,0.1005,5.1012,0f000001,0*ca3e42a8\n\tsystem status\tnormal 2 27.800000 0 0\trobot status\t95.753603\t124.155963\t8.007200\t-1.450873\t-0.189081\t-155.072886\t0.257000\t0.086000\n\t\n15:48:00.2\tlog_raw\tgps_raw\t#INSPVAXA,USB3,0,47.0,FINESTEERING,2107,283698.250,02000000,471d,15824;INS_ALIGNMENT_COMPLETE,INS_RTKFIXED,37.37124839401,126.72191465708,8.0076,22.3000,-0.0773,-0.2590,0.0230,-1.479636169,-0.110505972,244.843169403,0.4347,0.2979,0.5791,0.1126,0.0927,0.0785,0.0960,0.1005,5.1027,0f000001,0*0006d84b\n\tsystem status\tnormal 2 27.700000 0 0\trobot status\t95.624947\t124.102158\t8.007600\t-1.479636\t-0.110506\t-154.843169\t0.247000\t0.092000\n\t\n15:48:00.7\tlog_raw\tgps_raw\t#INSPVAXA,USB3,0,47.0,FINESTEERING,2107,283698.750,02000000,471d,15824;INS_ALIGNMENT_COMPLETE,INS_RTKFIXED,37.37124790607,126.72191317649,8.0096,22.3000,-0.0919,-0.2605,0.0162,-1.323665543,0.178775756,244.574454938,0.4347,0.2979,0.5791,0.1126,0.0927,0.0785,0.0960,0.1005,5.1027,0f000001,0*97fdd670\n\tsystem status\tnormal 2 27.800000 0 0\trobot status\t95.493799\t124.048006\t8.009600\t-1.323666\t0.178776\t-154.574455\t0.255000\t0.063000\n\t\n15:48:01.2\tlog_raw\tgps_raw\t#INSPVAXA,USB3,0,47.5,FINESTEERING,2107,283699.250,02000000,471d,15824;INS_ALIGNMENT_COMPLETE,INS_RTKFIXED,37.37124741280,126.72191168515,8.0116,22.3000,-0.0880,-0.2650,0.0236,-1.277654114,0.173050319,244.335495990,0.4352,0.2978,0.5791,0.1127,0.0927,0.0785,0.0959,0.1005,5.1036,0f000001,0*401d1919\n\tsystem status\tnormal 2 27.800000 0 0\trobot status\t95.361698\t123.993262\t8.011600\t-1.277654\t0.173050\t-154.335496\t0.326000\t-0.036000\n\t\n15:48:01.7\tlog_raw\tgps_raw\t#INSPVAXA,USB3,0,47.5,FINESTEERING,2107,283699.750,02000000,471d,15824;INS_ALIGNMENT_COMPLETE,INS_RTKFIXED,37.37124691977,126.72191021065,8.0139,22.3000,-0.0941,-0.2573,0.0260,-1.295740084,0.118148751,244.043765881,0.4352,0.2978,0.5791,0.1127,0.0927,0.0785,0.0959,0.1005,5.1036,0f000001,0*b4e001ab\n\tsystem status\tnormal 2 27.800000 0 0\trobot status\t95.231089\t123.938545\t8.013900\t-1.295740\t0.118149\t-154.043766\t0.366000\t-0.095000\n\t\n15:48:02.2\tlog_raw\tgps_raw\t#INSPVAXA,USB3,0,48.5,FINESTEERING,2107,283700.250,02000000,471d,15824;INS_ALIGNMENT_COMPLETE,INS_RTKFIXED,37.37124641299,126.72190870241,8.0157,22.3000,-0.0965,-0.2606,0.0330,-1.289006516,0.186517966,243.733079989,0.4358,0.2981,0.5791,0.1128,0.0927,0.0785,0.0959,0.1005,5.1040,0f000001,0*7b588f65\n\tsystem status\tnormal 2 27.700000 0 0\trobot status\t95.097492\t123.882302\t8.015700\t-1.289007\t0.186518\t-153.733080\t0.379000\t-0.108000\n\t\n15:48:02.7\tlog_raw\tgps_raw\t#INSPVAXA,USB3,0,48.5,FINESTEERING,2107,283700.750,02000000,471d,15824;INS_ALIGNMENT_COMPLETE,INS_RTKFIXED,37.37124591211,126.72190719117,8.0183,22.3000,-0.0934,-0.2790,0.0272,-1.230862677,0.124809038,243.414753616,0.4358,0.2981,0.5791,0.1128,0.0927,0.0785,0.0959,0.1005,5.1040,0f000001,0*24944499\n\tsystem status\tnormal 2 27.700000 0 0\trobot status\t94.963629\t123.826713\t8.018300\t-1.230863\t0.124809\t-153.414754\t0.243000\t0.106000\n\t\n15:48:03.2\tlog_raw\tgps_raw\t#INSPVAXA,USB3,0,48.0,FINESTEERING,2107,283701.250,02000000,471d,15824;INS_ALIGNMENT_COMPLETE,INS_RTKFIXED,37.37124542632,126.72190568049,8.0217,22.3000,-0.0782,-0.2571,0.0284,-0.983799928,0.018605262,242.857861412,0.4361,0.2983,0.5790,0.1125,0.0928,0.0785,0.0959,0.1004,5.1037,0f000001,0*579729be\n\tsystem status\tnormal 2 27.700000 0 0\trobot status\t94.829815\t123.772800\t8.021700\t-0.983800\t0.018605\t-152.857861\t0.262000\t0.105000\n\t\n15:48:03.7\tlog_raw\tgps_raw\t#INSPVAXA,USB3,0,48.0,FINESTEERING,2107,283701.750,02000000,471d,15824;INS_ALIGNMENT_COMPLETE,INS_RTKFIXED,37.37124504941,126.72190455554,8.0252,22.3000,-0.1066,-0.3087,0.0271,-0.874891899,0.189008715,240.527059520,0.4361,0.2983,0.5790,0.1125,0.0928,0.0785,0.0959,0.1004,5.1037,0f000001,0*9bbd18ba\n\tsystem status\tnormal 2 27.100000 0 0\trobot status\t94.730169\t123.730969\t8.025200\t-0.874892\t0.189009\t-150.527060\t0.325000\t0.146000\n\t\n15:48:04.2\tlog_raw\tgps_raw\t#INSPVAXA,USB3,0,50.5,FINESTEERING,2107,283702.250,02008000,471d,15824;INS_ALIGNMENT_COMPLETE,INS_RTKFIXED,37.37124442762,126.72190307020,8.0282,22.3000,-0.1382,-0.2404,0.0216,-0.866741092,0.060143860,235.368916733,0.4360,0.2989,0.5791,0.1125,0.0927,0.0785,0.0959,0.1004,5.1028,0f000001,0*0ab995b1\n\tsystem status\tnormal 2 27.200000 4 0\trobot status\t94.598600\t123.661962\t8.028200\t-0.866741\t0.060144\t-145.368917\t0.286000\t0.213000\n\t\n15:48:04.7\tlog_raw\tgps_raw\t#INSPVAXA,USB3,0,50.5,FINESTEERING,2107,283702.750,02008000,471d,15824;INS_ALIGNMENT_COMPLETE,INS_RTKFIXED,37.37124370430,126.72190170598,8.0314,22.3000,-0.1609,-0.2382,0.0230,-1.064164970,-0.109212362,230.360783935,0.4360,0.2989,0.5791,0.1125,0.0927,0.0785,0.0959,0.1004,5.1028,0f000001,0*391c17ea\n\tsystem status\tnormal 2 27.100000 4 0\trobot status\t94.477760\t123.581686\t8.031400\t-1.064165\t-0.109212\t-140.360784\t0.321000\t0.132000\n\t\n15:48:05.2\tlog_raw\tgps_raw\t#INSPVAXA,USB3,0,50.5,FINESTEERING,2107,283703.250,02008000,471d,15824;INS_ALIGNMENT_COMPLETE,INS_RTKFIXED,37.37124291299,126.72190041379,8.0333,22.3000,-0.1952,-0.2293,0.0238,-0.984755093,-0.132867348,225.970025862,0.4356,0.2991,0.5791,0.1126,0.0928,0.0785,0.0959,0.1003,5.0999,0f000001,0*698b4567\n\tsystem status\tnormal 2 27.200000 4 0\trobot status\t94.363300\t123.493864\t8.033300\t-0.984755\t-0.132867\t-135.970026\t0.306000\t0.142000\n\t\n15:48:05.7\tlog_raw\tgps_raw\t#INSPVAXA,USB3,0,50.5,FINESTEERING,2107,283703.750,02008000,471d,15824;INS_ALIGNMENT_COMPLETE,INS_RTKFIXED,37.37124204915,126.72189921350,8.0352,22.3000,-0.1844,-0.2111,0.0260,-0.917701758,-0.201673518,222.401686882,0.4356,0.2991,0.5791,0.1126,0.0928,0.0785,0.0959,0.1003,5.0999,0f000001,0*b00298a2\n\tsystem status\tnormal 2 27.200000 4 0\trobot status\t94.256980\t123.397992\t8.035200\t-0.917702\t-0.201674\t-132.401687\t0.294000\t0.105000\n\t\n15:48:06.2\tlog_raw\tgps_raw\t#INSPVAXA,USB3,0,52.5,FINESTEERING,2107,283704.250,02008000,471d,15824;INS_ALIGNMENT_COMPLETE,INS_RTKFIXED,37.37124115069,126.72189807141,8.0376,22.3000,-0.2004,-0.2048,0.0174,-1.022423432,-0.388489047,219.876868420,0.4350,0.2996,0.5792,0.1127,0.0932,0.0785,0.0959,0.1002,5.0962,0f000001,0*a3ed39a7\n\tsystem status\tnormal 2 27.200000 0 0\trobot status\t94.155815\t123.298278\t8.037600\t-1.022423\t-0.388489\t-129.876868\t0.306000\t0.089000\n\t\n15:48:06.7\tlog_raw\tgps_raw\t\tsystem status\tnormal 2 27.400000 0 0\trobot status\t94.056236\t123.194696\t8.039200\t-0.968680\t-0.555852\t-127.944433\t0.298000\t0.060000\n\t\n15:48:07.2\tlog_raw\tgps_raw\t\tsystem status\tnormal 2 27.500000 0 0\trobot status\t93.960092\t123.087665\t8.041400\t-1.035980\t-0.618606\t-126.611908\t0.305000\t0.036000\n\t\n15:48:07.7\tlog_raw\tgps_raw\t\tsystem status\tnormal 2 27.600000 0 0\trobot status\t93.866872\t122.980356\t8.044300\t-1.157794\t-0.594226\t-125.847764\t0.299000\t0.016000\n\t\n15:48:08.2\tlog_raw\tgps_raw\t#INSPVAXA,USB3,0,49.0,FINESTEERING,2107,283706.250,02000000,471d,15824;INS_ALIGNMENT_COMPLETE,INS_RTKFIXED,37.37123727449,126.72189373290,8.0459,22.3000,-0.2128,-0.1725,0.0234,-1.209481692,-0.641915990,215.491722437,0.4342,0.2996,0.5792,0.1131,0.0940,0.0785,0.0958,0.1000,5.0896,0f000001,0*17f33bf8\n\tsystem status\tnormal 2 27.700000 0 0\trobot status\t93.771517\t122.868084\t8.045900\t-1.209482\t-0.641916\t-125.491722\t0.251000\t0.054000\n\t\n15:48:08.7\tlog_raw\tgps_raw\t\tsystem status\tnormal 2 27.800000 0 0\trobot status\t93.675064\t122.755186\t8.047000\t-1.043283\t-0.673441\t-125.383196\t0.278000\t0.026000\n\t\n15:48:09.2\tlog_raw\tgps_raw\t\tsystem status\tnormal 2 27.800000 0 0\trobot status\t93.582390\t122.649376\t8.048600\t-0.778290\t-0.571414\t-125.533032\t0.293000\t-0.013000\n\t\n15:48:09.7\tlog_raw\tgps_raw\t\tsystem status\tnormal 2 27.800000 0 0\trobot status\t93.493987\t122.548763\t8.051100\t-0.480252\t-0.313792\t-125.614679\t0.301000\t-0.028000\n\t\n15:48:10.2\tlog_raw\tgps_raw\t\tsystem status\tnormal 2 27.800000 0 0\trobot status\t93.404974\t122.440860\t8.052000\t-0.744171\t-0.204031\t-125.840864\t0.300000\t-0.028000\n\t\n15:48:10.7\tlog_raw\tgps_raw\t#INSPVAXA,USB3,0,48.0,FINESTEERING,2107,283708.750,02000000,471d,15824;INS_ALIGNMENT_COMPLETE,INS_RTKFIXED,37.37123243346,126.72188856798,8.0524,22.3000,-0.2261,-0.1988,0.0348,-0.901144389,0.198517088,216.068250982,0.4339,0.3000,0.5792,0.1135,0.0940,0.0785,0.0956,0.0997,5.0860,0f000001,0*ba7ccbe0\n\tsystem status\tnormal 2 27.800000 0 0\trobot status\t93.314017\t122.330809\t8.052400\t-0.901144\t0.198517\t-126.068251\t0.299000\t-0.033000\n\t\n15:48:11.2\tlog_raw\tgps_raw\t#INSPVAXA,USB3,0,47.5,FINESTEERING,2107,283709.250,02000000,471d,15824;INS_ALIGNMENT_COMPLETE,INS_RTKFIXED,37.37123135236,126.72188744771,8.0521,22.3000,-0.2176,-0.2013,0.0343,-0.897424345,0.439323734,216.334218434,0.4339,0.3008,0.5792,0.1136,0.0941,0.0785,0.0955,0.0996,5.0867,0f000001,0*2487740e\n\tsystem status\tnormal 2 27.800000 0 0\trobot status\t93.214785\t122.210825\t8.052100\t-0.897424\t0.439324\t-126.334218\t0.313000\t-0.015000\n\t\n15:48:11.7\tlog_raw\tgps_raw\t\tsystem status\tnormal 2 27.800000 0 0\trobot status\t93.114632\t122.099079\t8.053300\t-0.104097\t0.205556\t-126.701117\t0.274000\t-0.074000
